vi "Arduino Write Log.vi"(8 "Arduino data":string, 9 "Command":string, 10 "Message":string, 11 "log ref":refnum<file>) -> ()   [LabVIEW 2021, in "FW Arduino Control.lvclass"]
uses:
  FW Arduino Control.lvclass
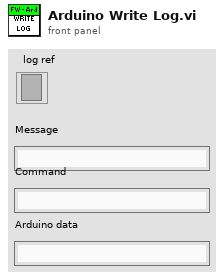
[diagram p1: front panel]
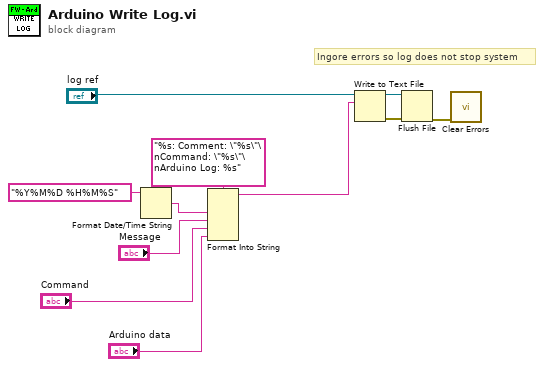
[diagram p0: block diagram]
diagram:
  # "Ingore errors so log does not stop system"
  n1 = Format Date/Time String(time format string (%c)="%Y%M%D %H%M%S") -> (date/time string=w5:string)  [unwired: 2 in]
  n2 = Format Into String(format string="%s: Comment: \"%s\"\nCommand: \"%s\"\nArduino Log: %s" ("time format string (%c)"), w5, "Message", "Command", "Arduino data") -> (resulting string=w2:string)  [unwired: 2 in, 1 out]
  n3 = Write to Text File(file (use dialog)="log ref", text=w2) -> (refnum out=w9:refnum<file>, error out=w11:errorcluster)  [unwired: 2 in, 1 out]
  n4 = Flush File(refnum=w9, error in=w11) -> (error out=w10:errorcluster)  [unwired: 1 out]
  n5 = call <vilib>:"Clear Errors.vi"("error in (no error)"=w10) -> ()  [unwired: 5 in, 2 out]
